vi "Drive for Distance FGV.vi"(7 "State":T1, 8 "error in":errorcluster, 11 "Desired Distance":dbl format="%#_13g") -> (0 "error out":errorcluster, 2 "Slow: Left (T) / Right (F)":bool, 3 "Complete?":bool)   [LabVIEW 2016]
doc: "FGV designed to allow you to drive for a set distance; only works in forward/backward orientation, cannot be used to turn."
uses:
  Drive for Distance States.ctl
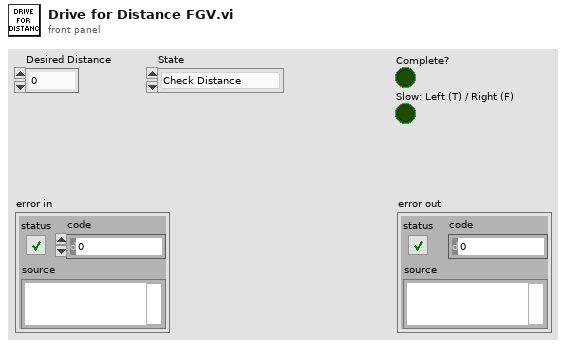
[diagram p1: front panel]
types:
  T1 = typedef "Drive for Distance States.ctl" = enum16{"Check Distance", "Initialize Distance"}
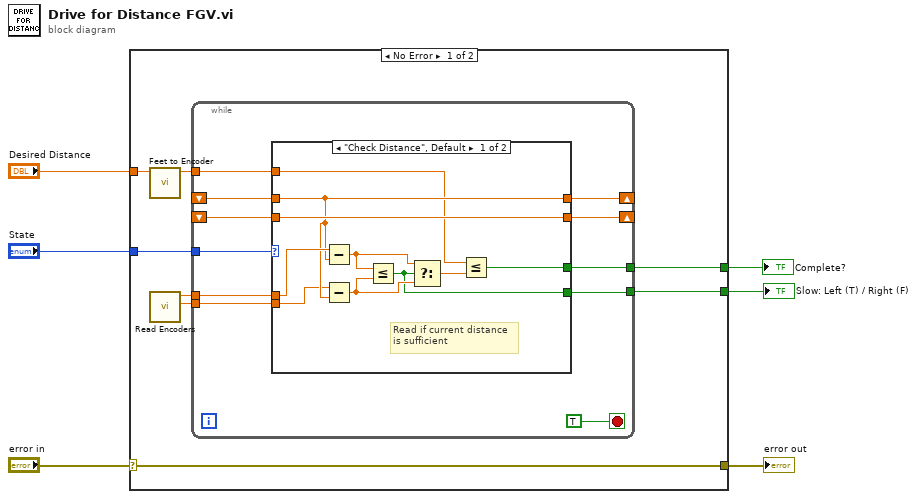
[diagram p0: block diagram]
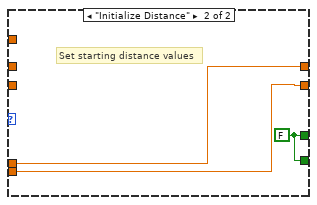
[diagram p2: hidden frame]
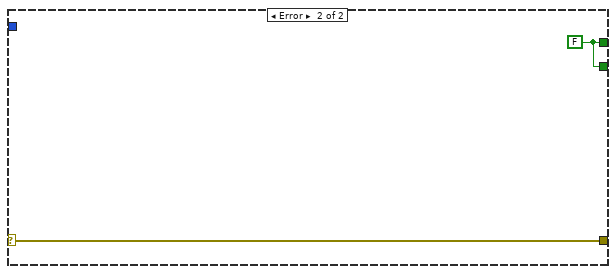
[diagram p3: hidden frame]
diagram:
  n1 = case shown="No Error" "error in" {
    selector: "error in" -> [w9 w40]
    tunnel: "State" -> [w14 _]
    tunnel: "Desired Distance" -> [w13 _]
    tunnel: [w10 w39] -> w4
    tunnel: [w9 w40] -> w2
    tunnel: [w7 w39] -> w1
    frame No Error {
      n2 = call "Feet to Encoder.vi"("Distance (ft)"=w13) -> ("Encoder Units"=w8:dbl)  [unwired: 10 in]
      n3 = call "Read Encoders.vi"() -> ("Right Encoder"=w11:dbl, "Left Encoder"=w12:dbl)  [unwired: 10 in]
      n4 = while {
        tunnel: w14 -> [w24]
        shift-right: [w23] -> _
        shift-left: _ -> [w21]
        shift-right: [w22] -> _
        shift-left: _ -> [w20]
        tunnel: w12 -> [w19]
        tunnel: w11 -> [w18]
        tunnel: w8 -> [w17]
        tunnel: [w16] -> w10
        tunnel: [w15] -> w7
        stop <- TRUE ("stop") stop-if-true
        n5 = case shown="\"Check Distance\", Default" w24 {
          tunnel: [w33 w38] -> w23
          tunnel: [w35 w37] -> w22
          tunnel: w21 -> [w33 _]
          tunnel: w20 -> [w35 _]
          tunnel: w19 -> [w34 w38]
          tunnel: w18 -> [w32 w37]
          tunnel: w17 -> [w28 _]
          tunnel: [w27 w36] -> w16
          tunnel: [w26 w36] -> w15
          frame "Check Distance", Default {
            # "Read if current distance\nis sufficient"
            n6 = Subtract(x=w34, y=w33) -> (x-y=w30:dbl)
            n7 = Subtract(x=w32, y=w33) -> (x-y=w31:dbl)
            n8 = Less Or Equal?(x=w30, y=w31) -> (x <= y?=w26:bool)
            n9 = Select(t=w30, s=w26, f=w31) -> (s? t:f=w29:dbl)
            n10 = Less Or Equal?(x=w28, y=w29) -> (x <= y?=w27:bool)
          }
          frame "Initialize Distance" {
            w36 = FALSE
            # "Set starting distance values"
          }
        }
      }
    }
    frame Error {
      w39 = FALSE
    }
  }
  "Complete?" <- w4
  "error out" <- w2
  "Slow: Left (T) / Right (F)" <- w1
